vi "Array difference.vi"(8 "error in (no error)":errorcluster, 9 "Channels Array 2":T1, 10 "Channels Array":T1) -> (0 "error out":errorcluster, 1 "Array 2-(array1&2)":T1, 2 "Array 1-(array1&2)":T1)   [LabVIEW 2016, in "pickering.lvclass"]
uses:
  pickering.lvclass
  Typedefs/Channels-Array.ctl
  Typedefs/Channel-Cluster.ctl
  Typedefs/ChannelX-ComboBox.ctl
  Typedefs/ChannelY-ComboBox.ctl
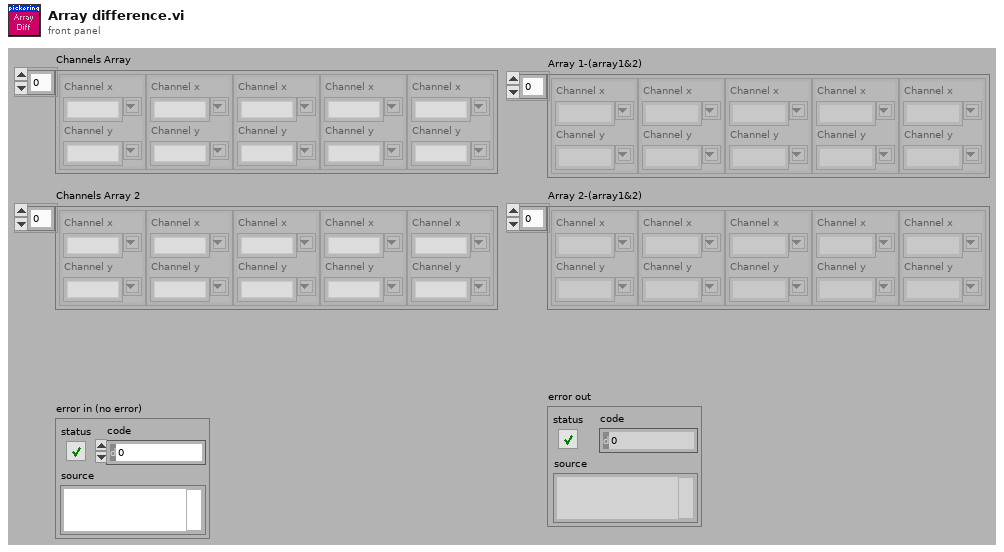
[diagram p1: front panel]
types:
  T1 = typedef "pickering.lvclass/Channels-Array.ctl" = T2[]
  T2 = typedef "pickering.lvclass/Channel-Cluster.ctl" = cluster{"Channel x":T3, "Channel y":T4}
  T3 = typedef "pickering.lvclass/ChannelX-ComboBox.ctl" = string
  T4 = typedef "pickering.lvclass/ChannelY-ComboBox.ctl" = string
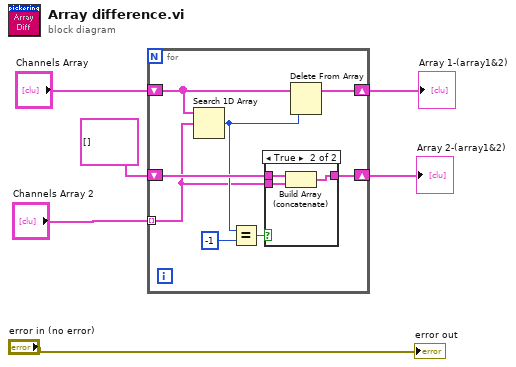
[diagram p0: block diagram]
diagram:
  n1 = for {
    tunnel: "Channels Array 2" -> [w7] mode=indexing
    shift-right: [w14] -> w5
    shift-left: "Channels Array" -> [w10]
    shift-right: [w13] -> w3
    shift-left: cluster{"String":string, "String 2":string}[] [] -> [w9]
    n2 = Search 1D Array(1D array=w10, element=w7) -> (index of element=w8:i32)  [unwired: 1 in]
    n3 = Equal?(x=w8, y=-1) -> (x = y?=w12:bool)
    n4 = case shown="True" w12 {
      tunnel: w7 -> [_ w18]
      tunnel: [w15 w17] -> w13
      tunnel: w9 -> [w15 w16]
      frame False {
      }
      frame True {
        n5 = Build Array (concatenate)(w16, w18) -> (w17:T2[])
      }
    }
    n6 = Delete From Array(array=w10, index=w8) -> (array with subset deleted=w14:T1)  [unwired: 1 in, 1 out]
  }
  "Array 1-(array1&2)" <- w5
  "Array 2-(array1&2)" <- w3
  "error out" <- "error in (no error)"
